vi "RateScan_Javi.vi"(0 "ftHandle_in":u32, 5 "VISA resource name":refnum<visa-resource-name>="USB0::0x0957::0x4108::MY51400415::INSTR", 7 "Path":path, 9 "String":string, 11 "error in (no error)":errorcluster) -> (4 "ftHandle_out":u32, 6 "VISA resource name out":refnum<visa-resource-name>, 15 "error out":errorcluster)   [LabVIEW 2019]
uses:
  Global_STOP.vi
  Library VI/Global.Salir Ya.vi
panel:
  out "B 2":u8(slide)=9 scale=0.0..100.0
  out "% 2":u8=9 format="%02d%%"
  out "Indicador 2":string="VTheo 0,0500V (Vreal 0,0000V)\nChannel 7 Adder C\nTotal Errors: 0"
  out "HLTHx 3":dbl
  out "DAC TH0,TH1,TH2 3":u16
  out "LLTHx 3":dbl
  out "DAC TH3,TH4,TH5 3":u16
  out "Reference 2":T1={"Sumador"=2, "Canal"=6, "Tension"=0, "Tension Real"=0.0}
  out "Amplitude 2":dbl
  out "B":u8(slide)=9 scale=0.0..100.0
  out "%":u8=9 format="%02d%%"
  out "Indicador":string="VTheo 0,0500V (Vreal 0,0000V)\nChannel 7 Adder C\nTotal Errors: 0"
  out "HLTHx 2":dbl
  out "DAC TH0,TH1,TH2 2":u16
  out "LLTHx 2":dbl
  out "DAC TH3,TH4,TH5 2":u16
  out "Reference":T1={"Sumador"=2, "Canal"=6, "Tension"=0, "Tension Real"=0.0}
  out "Amplitude":dbl
  out "EJECUTANDO TEST SUMADORES":u8(slide) scale=0.0..10.0
  out "Flag_programoPulso":bool
  out "spreadsheet string":string
  out "TOTAL VALORES LLTHX":dbl[][](array[numeric])
  out "Array":u16[](array[numeric])
  out "x*y":u32
  out "TOTAL VALORES HLTHX":dbl[][](array[numeric])
  out "Valor Asic":u16 format="%x"
  out "TOTAL VALORES":u16[][](array[numeric]) format="%x"
  out "DAC TH3,TH4,TH5":u16
  out "LLTHx":dbl
  out "DAC TH0,TH1,TH2":u16
  out "HLTHx":dbl
  # "IN"
  # "1 + 2 + 3"
  # "ADC"
  # "ADC"
  # "Vin Asic"
  # "Vin Asic"
  # "ADD A/1"
  # "ADD B/1"
  # "ADD C/1"
  # "ADD A/0"
  # "ADD B/0"
  # "ADD C/0"
  # "50mV"
  # "50mV"
  # "90mV"
  # "90mV"
  # "130mV"
  # "130mV"
  # "170mV"
  # "170mV"
  # "210mV"
  # "210mV"
  # "250mV"
  # "250mV"
  # "290mV"
  # "290mV"
  # "330mV"
  # "330mV"
  # "370mV"
  # "370mV"
  # "410mV"
  # "410mV"
  # "TH0"
  # "TH1"
  # "TH2"
  # "DAC"
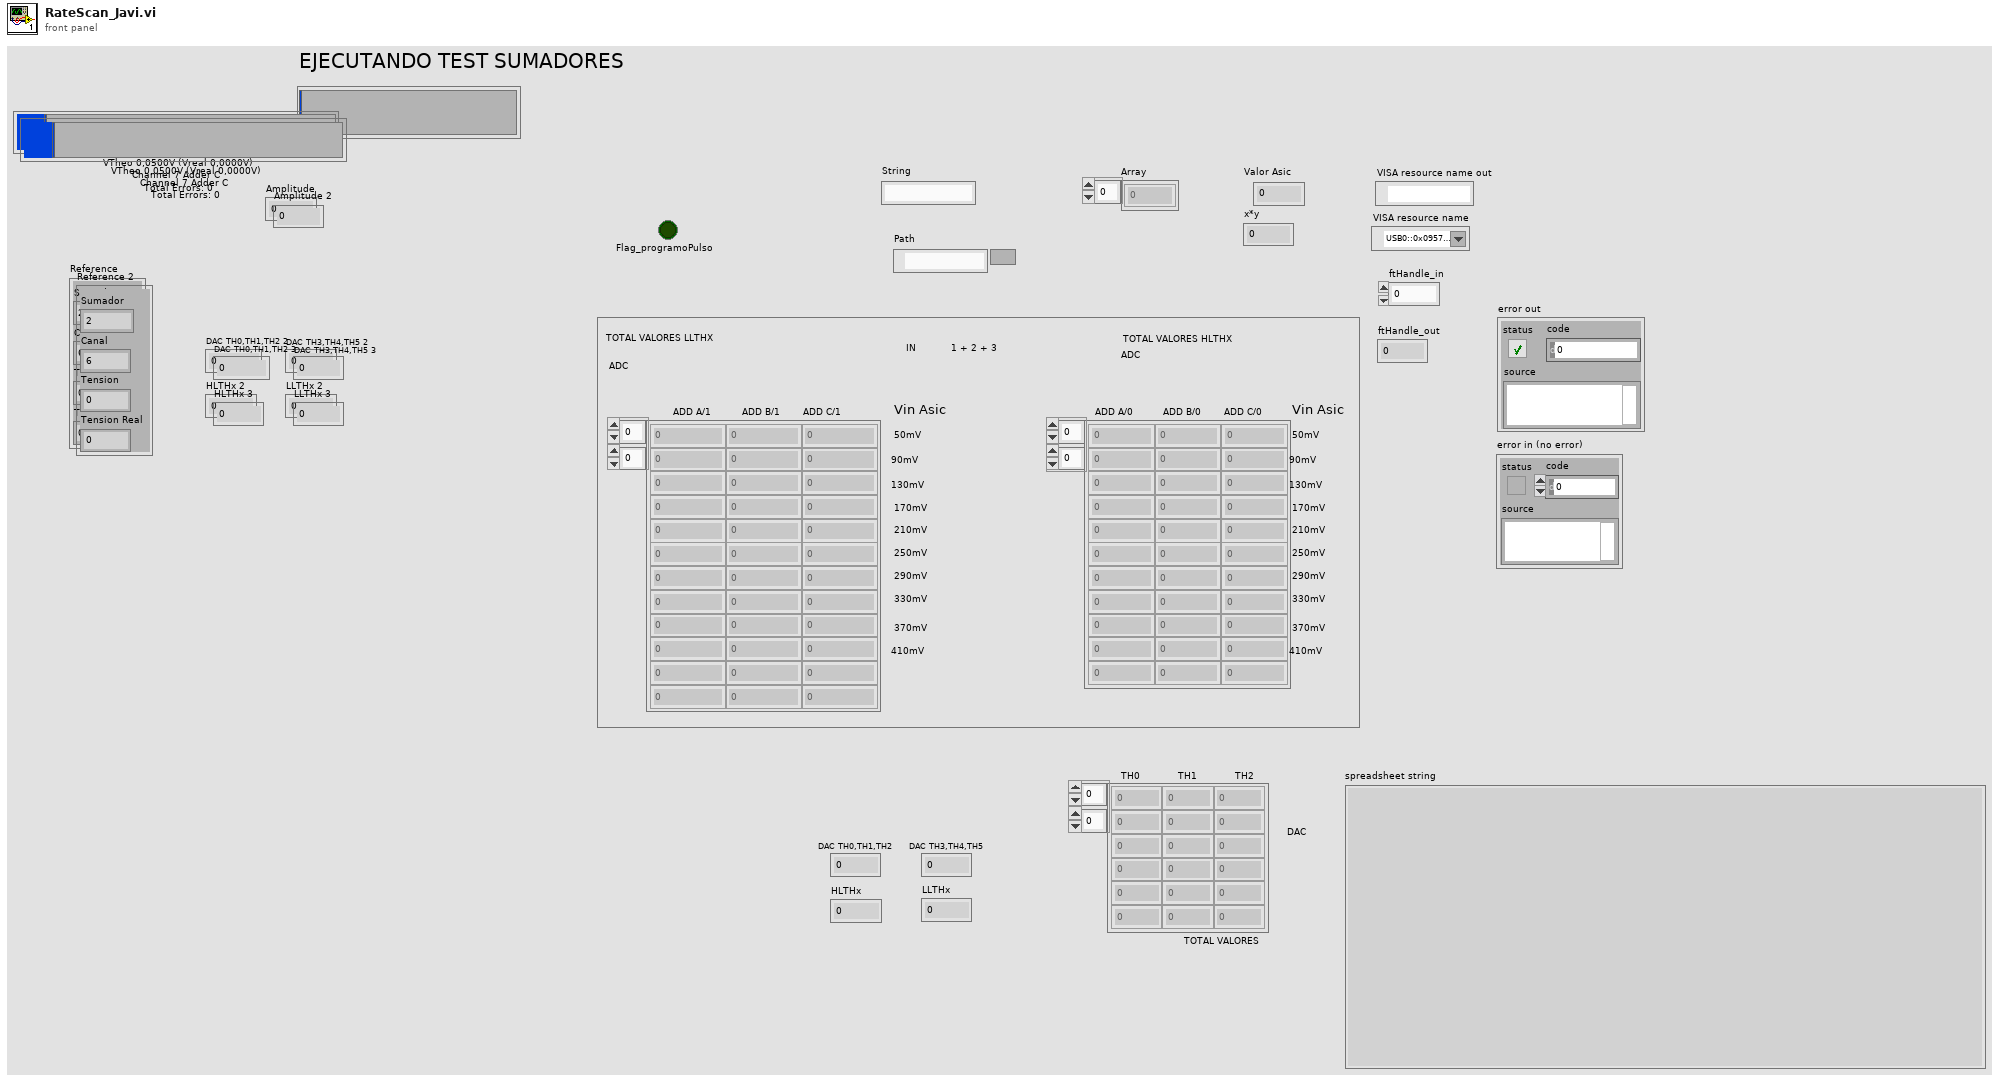
[diagram p1: front panel]
types:
  T1 = cluster{"Sumador":u8, "Canal":u8, "Tension":u8, "Tension Real":dbl}
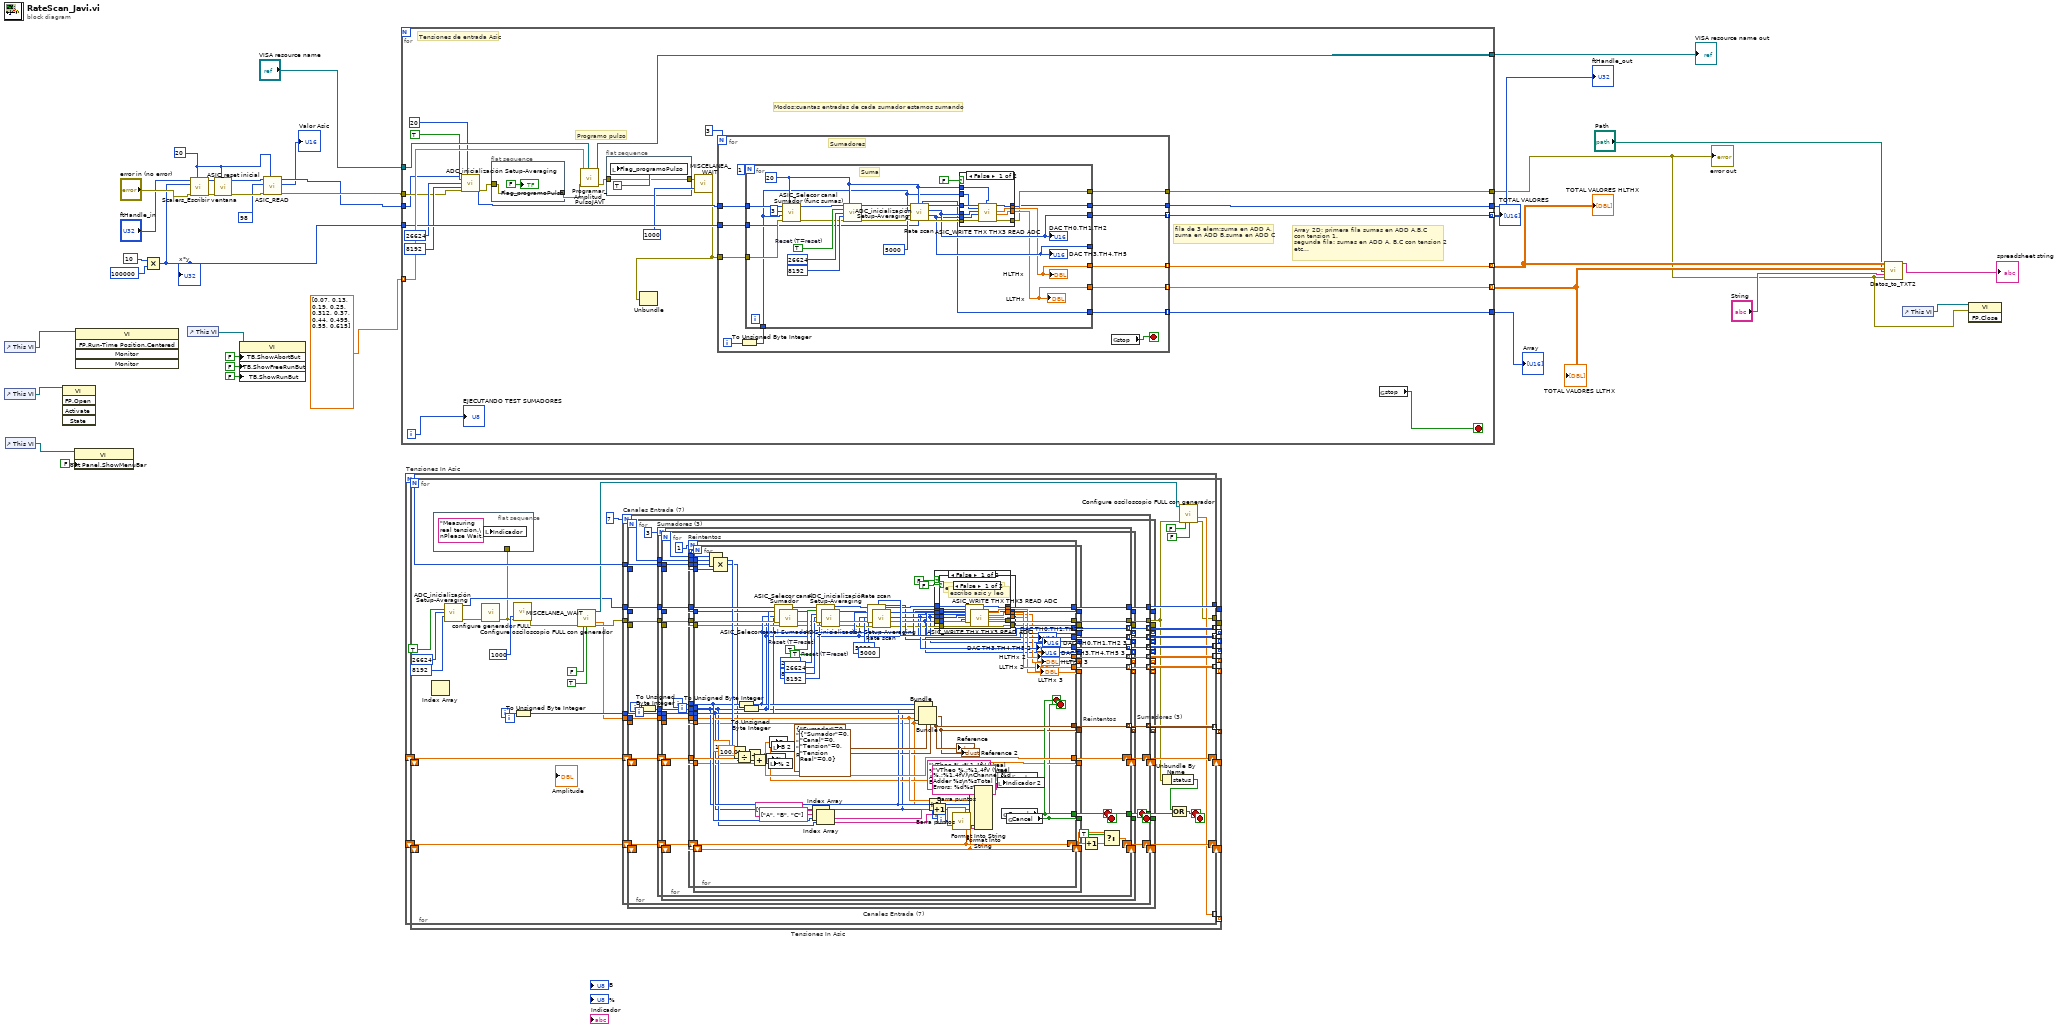
[diagram p0: block diagram]
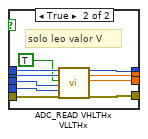
[diagram p2: hidden frame]
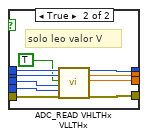
[diagram p3: hidden frame]
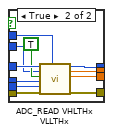
[diagram p4: hidden frame]
diagram:
  w18 = u32 20 ("Espera acceso USB")
  n1 = control-ref of="This VI"() -> (w10:refnum<vi>)
  n2 = control-ref of="This VI"() -> (w7:refnum<vi>)
  n3 = control-ref of="This VI"() -> (w6:refnum<vi>)
  n4 = invoke class="VI" method="FP.Open"(reference=w7) -> ()  [unwired: 4 in, 5 out]
  n5 = property class="VI"(reference=w6, "Front Panel.ShowMenuBar"=FALSE ("Front Panel Window:Show Menu Bar")) -> ()  [unwired: 1 in, 2 out]
  n6 = invoke class="VI" method="FP.Run-Time Position.Centered"(reference=w10) -> ()  [unwired: 4 in, 5 out]
  n7 = Multiply(x=u32 10 ("Ventana"), y=u32 100000 ("Ventana")) -> (x*y=w28:u32)
  "x*y" <- w28
  n8 = control-ref of="This VI"() -> (w4:refnum<vi>)
  n9 = call "Scalers_Escribir ventana.vi"("Espera acceso USB"=w18, "error in"="error in (no error)", "Ventana"=w28, "ftHandle_in"="ftHandle_in") -> ("error out"=w33:errorcluster, "ftHandle_out"=w32:u32)  [unwired: 6 in]
  n10 = call "ASIC_reset inicial.vi"("Espera acceso USB"=w18, "error in"=w33, "ftHandle_in"=w32) -> ("error out"=w23:errorcluster, "ftHandle_out"=w24:u32)  [unwired: 7 in]
  n11 = property class="VI"(reference=w4, "TB.ShowAbortBut"=FALSE ("Tool Bar:Show Abort Button"), "TB.ShowFreeRunBut"=FALSE ("Tool Bar:Show Free Run Button"), "TB.ShowRunBut"=FALSE ("Tool Bar:Show Run Button")) -> ()  [unwired: 1 in, 2 out]
  n12 = call "ASIC_READ.vi"("Espera acceso USB"=w18, "error in"=w23, "Direccion Registro Asic"=u8 98, "ftHandle_in"=w24) -> ("error out"=w22:errorcluster, "Valor Asic"=→"Valor Asic":u16, "ftHandle_out"=w21:u32)  [unwired: 5 in]
  n13 = for {
    tunnel: dbl[] [0.07, 0.13, 0.19, 0.25, 0.312, 0.37, 0.44, 0.495, 0.55, 0.615] -> [w61] mode=indexing
    tunnel: "VISA resource name" -> [w60]
    tunnel: w21 -> [w47]
    tunnel: w22 -> [w49]
    tunnel: w28 -> [w59]
    tunnel: [w58] -> w8
    tunnel: [w57] -> w27
    tunnel: [w56] -> w26
    tunnel: [w55] -> w25 mode=indexing
    tunnel: [w54] -> w17
    tunnel: [w44] -> w15 mode=indexing
    tunnel: [w43] -> w14 mode=indexing
    i -> [w36]
    stop <- w37 stop-if-true
    # "fila de 3 elem:suma en ADD A,\nsuma en ADD B,suma en ADD C"
    # "Modos:cuantas entradas de cada sumador estamos sumando"
    # "Array 2D: primera fila sumas en ADD A,B,C\ncon tension 1.\nsegunda fila: sumas en ADD A, B,C con tension 2\netc..."
    # "Programo pulso"
    # "Tensiones de entrada Asic"
    n14 = call "ADC_inicialización Setup-Averaging.vi"("ftHandle_in 2"=w47, "Espera acceso USB"=u32 20, "Reset (T=reset)"=TRUE, "Registro Setup (0x6800)"=u16 26624, "Registro Averaging (0x3200)"=u16 8192 ("Registro Setup (0x6800)"), "error in 2"=w49) -> ("ftHandle_out"=w46:u32, "error out"=w41:errorcluster)  [unwired: 8 in]
    n15 = flat-sequence {
      tunnel: [w65] -> w40
      tunnel: w41 -> [w65]
      frame #0 {
        "Flag_programoPulso" <- FALSE ("Flag_programoPulso")
      }
    }
    n16 = call "Programar_Amplitud_PulsoJAVI.vi"("error in (no error)"=w40, "Numeric"=w61, "VISA Refnum in"=w60) -> ("Error OUT"=w39:errorcluster, "VISA resource name out"=w57:refnum<visa-resource-name>)  [unwired: 7 in]
    n17 = flat-sequence {
      tunnel: w39 -> [w62]
      tunnel: [w62] -> w38
      frame #0 {
        n18 = local write "Flag_programoPulso"(TRUE ("Flag_programoPulso")) -> ()
      }
    }
    n19 = call "MISCELANEA_WAIT.vi"("ms wait IN"=u32 1000, "Error IN"=w38) -> ("Error OUT"=w42:errorcluster)  [unwired: 16 in, 1 out]
    n20 = Unbundle(w42) -> ()  [unwired: 3 out]
    n21 = for {
      N: 3 -> [_]
      tunnel: w46 -> [w77]
      tunnel: w42 -> [w74]
      tunnel: w59 -> [w73]
      tunnel: [w72] -> w55 mode=indexing
      tunnel: [w71] -> w58
      tunnel: [w70] -> w56
      tunnel: [w69] -> w54 mode=indexing
      tunnel: [w68] -> w44 mode=indexing
      tunnel: [w67] -> w43 mode=indexing
      i -> [w76]
      stop <- w66 stop-if-true
      # "Sumadores"
      n22 = To Unsigned Byte Integer(number=w76) -> (unsigned 8bit integer=w75:u8)
      n23 = for {
        N: 1 -> [_]
        tunnel: w77 -> [w91]
        tunnel: w75 -> [w80]
        tunnel: w74 -> [w90]
        tunnel: w73 -> [w88]
        tunnel: [w87] -> w72
        tunnel: [w86] -> _
        tunnel: [w85] -> w68
        tunnel: [w84] -> w67
        tunnel: [w83] -> w71
        tunnel: [w82] -> w69
        tunnel: [w81] -> w70
        w89 = u32 20 ("Espera acceso USB")
        w102 = TRUE  # Reset (T=reset)
        # "Suma"
        n24 = call "ASIC_Selecor canal Sumador (func sumas).vi"("Espera acceso USB"=w89, "error in"=w90, "Sumador"=w80, "Modo"=u8 3, "ftHandle_in"=w91) -> ("error out"=w97:errorcluster, "ftHandle_out"=w94:u32)  [unwired: 3 in, 2 out]
        n25 = call "ADC_inicialización Setup-Averaging.vi"("ftHandle_in 2"=w94, "Espera acceso USB"=w89, "Reset (T=reset)"=w102, "Registro Setup (0x6800)"=u16 26624, "Registro Averaging (0x3200)"=u16 8192 ("Registro Setup (0x6800)"), "error in 2"=w97) -> ("ftHandle_out"=w99:u32, "error out"=w98:errorcluster)  [unwired: 8 in]
        n26 = call "Rate scan.vi"("T Ventana"=w88, "Espera acceso USB"=w89, "error in 2"=w98, "Valor buscado scalers (5000)"=u16 5000 ("Valor buscado scalers"), "Sumador"=w80, "ftHandle_in 2"=w99) -> ("error out 2"=w95:errorcluster, "DAC\nTH3,TH4,TH5"=w86:u16, "DAC\nTH0,TH1,TH2"=w87:u16, "ftHandle_out 2"=w96:u32, "Scaler 1"=w82:u16)  [unwired: 1 in]
        "DAC TH0,TH1,TH2" <- w87
        "DAC TH3,TH4,TH5" <- w86
        n27 = case shown="False" FALSE {
          tunnel: w96 -> [w112 w123]
          tunnel: w95 -> [w109 w122]
          tunnel: [w107 w121] -> w81
          tunnel: [w108 w120] -> w83
          tunnel: [w106 w119] -> w85
          tunnel: [w105 w118] -> w84
          tunnel: w87 -> [w111 w117]
          tunnel: w86 -> [w110 w116]
          tunnel: w89 -> [w104 w114]
          tunnel: w80 -> [w103 w113]
          frame False {
            n28 = call "ASIC_WRITE THX THX3 READ ADC.vi"("ftHandle_in"=w112, "Sumador"=w103, "THX"=w111, "THX+3"=w110, "error in"=w109, "Espera acceso USB 2"=w104) -> ("ftHandle_out"=w107:u32, "HLTHx"=w106:dbl, "LLTHx"=w105:dbl, "error out"=w108:errorcluster)  [unwired: 10 in]
          }
          frame True {
            n29 = call "ADC_READ VHLTHx VLLTHx.vi"("ftHandle_out 2"=w123, "Sumador"=w113, "referenciar"=TRUE, "ref DAC\nTH0,TH1,TH2"=w117, "ref DAC\nTH3,TH4,TH5"=w116, "error out 2"=w122, "Espera acceso FT"=w114) -> ("ftHandle_out"=w121:u32, "HLTHx"=w119:dbl, "LLTHx"=w118:dbl, "error out"=w120:errorcluster)  [unwired: 9 in]
          }
        }
        "HLTHx" <- w85
        "LLTHx" <- w84
      }
      n30 = global read "Global_STOP.vi" "stop"() -> (w66:bool)
    }
    n31 = global read "Global_STOP.vi" "stop"() -> (w37:bool)
    "EJECUTANDO TEST SUMADORES" <- w36
  }
  "error out" <- w8
  "VISA resource name out" <- w27
  "ftHandle_out" <- w26
  "TOTAL VALORES" <- w25
  "TOTAL VALORES HLTHX" <- w15
  "Array" <- w17
  "TOTAL VALORES LLTHX" <- w14
  n32 = for "Tensiones In Asic" {
    N -> [w146]
    tunnel: [w157] -> _ mode=indexing
    tunnel: [w156] -> _ mode=indexing
    tunnel: [w152] -> _ mode=indexing
    tunnel: [w151] -> _ mode=indexing
    tunnel: [w149] -> _ mode=indexing
    tunnel: [w147] -> _ mode=indexing
    shift-right: [w144] -> _
    shift-left: _ -> [w145]
    shift-right: [w142] -> _
    shift-left: _ -> [w143]
    tunnel: [w158] -> _
    tunnel: [w135] -> _
    tunnel: [w136] -> _ mode=indexing
    i -> [w150]
    stop <- w127 stop-if-true
    n33 = Index Array() -> ()  [unwired: 2 in, 1 out]
    n34 = flat-sequence {
      tunnel: w124 -> [_]
      frame #0 {
        n35 = local write "Indicador"("Measuring real tension.\nPlease Wait." ("Indicador")) -> ()
      }
    }
    n36 = call "ADC_inicialización Setup-Averaging.vi"("Reset (T=reset)"=TRUE, "Registro Setup (0x6800)"=u16 26624, "Registro Averaging (0x3200)"=u16 8192 ("Registro Setup (0x6800)")) -> ("ftHandle_out"=w126:u32, "error out"=w125:errorcluster)  [unwired: 11 in]
    n37 = call "configure generador FULL.vi"("error in"=w125) -> ("error out"=w124:errorcluster)  [unwired: 8 in, 2 out]
    n38 = call "MISCELANEA_WAIT.vi"("ms wait IN"=u32 1000, "Error IN"=w124) -> ("Error OUT"=w140:errorcluster)  [unwired: 16 in, 1 out]
    n39 = To Unsigned Byte Integer(number=w150) -> (unsigned 8bit integer=w148:u8)
    n40 = call "Configure osciloscopio FULL con generador.vi"("error out"=w140, "Esperar a completar estadisticas"=FALSE ("Wait medida"), "Configurar Osciloscopio"=TRUE ("Solo Medida")) -> ("VISA resource name out 2"=w131:refnum<visa-resource-name>, "Math (CH1-CH2)"=w137:dbl, "error out 2"=w139:errorcluster)  [unwired: 8 in, 2 out]
    n41 = for "Canales Entrada (7)" {
      N: 7 -> [w167]
      tunnel: [w175] -> w157 mode=indexing
      tunnel: [w174] -> w156 mode=indexing
      tunnel: [w173] -> w152 mode=indexing
      tunnel: [w172] -> w151 mode=indexing
      tunnel: w148 -> [w171]
      tunnel: w137 -> [w170]
      tunnel: [w169] -> w149 mode=indexing
      tunnel: [w168] -> w147 mode=indexing
      tunnel: w146 -> [w166]
      shift-right: [w164] -> w144
      shift-left: w145 -> [w165]
      tunnel: [w163] -> w128
      shift-right: [w161] -> w142
      shift-left: w143 -> [w162]
      tunnel: w126 -> [w182]
      tunnel: [w177] -> w158
      tunnel: w139 -> [w181]
      tunnel: [w176] -> w130
      i -> [w180]
      stop <- w163 stop-if-true
      n42 = To Unsigned Byte Integer(number=w180) -> (unsigned 8bit integer=w178:u8)
      n43 = for "Sumadores (3)" {
        N: 3 -> [w200]
        tunnel: w178 -> [w196]
        tunnel: [w208] -> w175 mode=indexing
        tunnel: [w207] -> w174 mode=indexing
        tunnel: [w192] -> w173 mode=indexing
        tunnel: [w191] -> w172 mode=indexing
        tunnel: w171 -> [w201]
        tunnel: w170 -> [w197]
        tunnel: [w203] -> w169 mode=indexing
        tunnel: [w202] -> w168 mode=indexing
        tunnel: w167 -> [w199]
        tunnel: w166 -> [w198]
        shift-right: [w193] -> w164
        shift-left: w165 -> [w194]
        tunnel: [w188] -> w163
        shift-right: [w187] -> w161
        shift-left: w162 -> [w189]
        tunnel: w182 -> [w205]
        tunnel: [w204] -> w177
        tunnel: w181 -> [w206]
        tunnel: [w183] -> w176
        i -> [w195]
        stop <- w188 stop-if-true
        n44 = for "Reintentos" {
          N: 1 -> [_]
          tunnel: [w215] -> w208
          tunnel: [w214] -> w207
          tunnel: w205 -> [w249]
          tunnel: [w246] -> w204
          tunnel: [w243] -> w203
          tunnel: [w242] -> w202
          tunnel: w201 -> [w221]
          tunnel: w200 -> [w240]
          tunnel: w199 -> [w239]
          tunnel: w198 -> [w238]
          tunnel: w197 -> [w209]
          tunnel: w196 -> [w212]
          tunnel: w195 -> [w234]
          tunnel: [w210] -> w188
          tunnel: [w226] -> w192
          tunnel: [w225] -> w191
          tunnel: w194 -> [w229]
          tunnel: [w227] -> w193
          shift-right: [w222] -> w186
          shift-left: w189 -> [w222]
          tunnel: w206 -> [w250]
          tunnel: [w245] -> w183
          i -> [w224]
          stop <- w210 stop-if-true
          w252 = TRUE  # Reset (T=reset)
          n45 = for "Tensiones In Asic" {
            N -> [w275]
            tunnel: [w286] -> _ mode=indexing
            tunnel: [w285] -> _ mode=indexing
            tunnel: [w281] -> _ mode=indexing
            tunnel: [w280] -> _ mode=indexing
            tunnel: [w278] -> _ mode=indexing
            tunnel: [w276] -> _ mode=indexing
            shift-right: [w273] -> _
            shift-left: _ -> [w274]
            shift-right: [w271] -> _
            shift-left: _ -> [w272]
            tunnel: [w287] -> _
            tunnel: [w264] -> _
            tunnel: [w265] -> _ mode=indexing
            i -> [w279]
            stop <- w256 stop-if-true
            n46 = Index Array() -> ()  [unwired: 2 in, 1 out]
            n47 = flat-sequence {
              tunnel: w253 -> [_]
              frame #0 {
                n48 = local write "Indicador 2"("Measuring real tension.\nPlease Wait." ("Indicador")) -> ()
              }
            }
            n49 = call "ADC_inicialización Setup-Averaging.vi"("Reset (T=reset)"=TRUE, "Registro Setup (0x6800)"=u16 26624, "Registro Averaging (0x3200)"=u16 8192 ("Registro Setup (0x6800)")) -> ("ftHandle_out"=w255:u32, "error out"=w254:errorcluster)  [unwired: 11 in]
            n50 = call "configure generador FULL.vi"("error in"=w254) -> ("error out"=w253:errorcluster)  [unwired: 8 in, 2 out]
            n51 = call "MISCELANEA_WAIT.vi"("ms wait IN"=u32 1000, "Error IN"=w253) -> ("Error OUT"=w269:errorcluster)  [unwired: 16 in, 1 out]
            n52 = To Unsigned Byte Integer(number=w279) -> (unsigned 8bit integer=w277:u8)
            n53 = call "Configure osciloscopio FULL con generador.vi"("error out"=w269, "Esperar a completar estadisticas"=FALSE ("Wait medida"), "Configurar Osciloscopio"=TRUE ("Solo Medida")) -> ("VISA resource name out 2"=w260:refnum<visa-resource-name>, "Math (CH1-CH2)"=w266:dbl, "error out 2"=w268:errorcluster)  [unwired: 8 in, 2 out]
            n54 = for "Canales Entrada (7)" {
              N: 7 -> [w296]
              tunnel: [w304] -> w286 mode=indexing
              tunnel: [w303] -> w285 mode=indexing
              tunnel: [w302] -> w281 mode=indexing
              tunnel: [w301] -> w280 mode=indexing
              tunnel: w277 -> [w300]
              tunnel: w266 -> [w299]
              tunnel: [w298] -> w278 mode=indexing
              tunnel: [w297] -> w276 mode=indexing
              tunnel: w275 -> [w295]
              shift-right: [w293] -> w273
              shift-left: w274 -> [w294]
              tunnel: [w292] -> w257
              shift-right: [w290] -> w271
              shift-left: w272 -> [w291]
              tunnel: w255 -> [w311]
              tunnel: [w306] -> w287
              tunnel: w268 -> [w310]
              tunnel: [w305] -> w259
              i -> [w309]
              stop <- w292 stop-if-true
              n55 = To Unsigned Byte Integer(number=w309) -> (unsigned 8bit integer=w307:u8)
              n56 = for "Sumadores (3)" {
                N: 3 -> [w329]
                tunnel: w307 -> [w325]
                tunnel: [w337] -> w304 mode=indexing
                tunnel: [w336] -> w303 mode=indexing
                tunnel: [w321] -> w302 mode=indexing
                tunnel: [w320] -> w301 mode=indexing
                tunnel: w300 -> [w330]
                tunnel: w299 -> [w326]
                tunnel: [w332] -> w298 mode=indexing
                tunnel: [w331] -> w297 mode=indexing
                tunnel: w296 -> [w328]
                tunnel: w295 -> [w327]
                shift-right: [w322] -> w293
                shift-left: w294 -> [w323]
                tunnel: [w317] -> w292
                shift-right: [w316] -> w290
                shift-left: w291 -> [w318]
                tunnel: w311 -> [w334]
                tunnel: [w333] -> w306
                tunnel: w310 -> [w335]
                tunnel: [w312] -> w305
                i -> [w324]
                stop <- w317 stop-if-true
                n57 = for "Reintentos" {
                  N: 1 -> [_]
                  tunnel: [w344] -> w337
                  tunnel: [w343] -> w336
                  tunnel: w334 -> [w378]
                  tunnel: [w375] -> w333
                  tunnel: [w372] -> w332
                  tunnel: [w371] -> w331
                  tunnel: w330 -> [w350]
                  tunnel: w329 -> [w369]
                  tunnel: w328 -> [w368]
                  tunnel: w327 -> [w367]
                  tunnel: w326 -> [w338]
                  tunnel: w325 -> [w341]
                  tunnel: w324 -> [w363]
                  tunnel: [w339] -> w317
                  tunnel: [w355] -> w321
                  tunnel: [w354] -> w320
                  tunnel: w323 -> [w358]
                  tunnel: [w356] -> w322
                  shift-right: [w351] -> w315
                  shift-left: w318 -> [w351]
                  tunnel: w335 -> [w379]
                  tunnel: [w374] -> w312
                  i -> [w353]
                  stop <- w339 stop-if-true
                  w381 = TRUE  # Reset (T=reset)
                  n58 = Compound Arithmetic op=MULTIPLY(w369, w368, w367) -> (w366:i32)
                  n59 = Divide(x=100.0, y=w366) -> (x/y=w357:dbl)
                  n60 = To Unsigned Byte Integer(number=w363) -> (unsigned 8bit integer=w340:u8)
                  n61 = Add(x=w357, y=w358) -> (x+y=w356:dbl)
                  n62 = local write "% 2"(w356) -> ()
                  n63 = local write "B 2"(w356) -> ()
                  n64 = call "ASIC_Selecor canal Sumador.vi"("error in"=w379, "Sumador"=w340, "Canal"=w341, "ftHandle_in"=w378) -> ("error out"=w377:errorcluster, "ftHandle_out"=w376:u32)  [unwired: 5 in, 1 out]
                  n65 = Index Array(array=string[] ["A", "B", "C"], index=w363) -> (element=w362:string)
                  n66 = call "ADC_inicialización Setup-Averaging.vi"("ftHandle_in 2"=w376, "Reset (T=reset)"=w381, "Registro Setup (0x6800)"=u16 26624, "Registro Averaging (0x3200)"=u16 8192 ("Registro Setup (0x6800)"), "error in 2"=w377) -> ("ftHandle_out"=w349:u32, "error out"=w348:errorcluster)  [unwired: 9 in]
                  n67 = call "Rate scan.vi"("error in 2"=w348, "Valor buscado scalers (5000)"=u16 5000 ("Valor buscado scalers"), "Sumador"=w340, "ftHandle_in 2"=w349) -> ("error out 2"=w346:errorcluster, "DAC\nTH3,TH4,TH5"=w343:u16, "DAC\nTH0,TH1,TH2"=w344:u16, "ftHandle_out 2"=w347:u32, "Scaler 1"=w372:u16)  [unwired: 3 in]
                  "DAC TH0,TH1,TH2 3" <- w344
                  "DAC TH3,TH4,TH5 3" <- w343
                  n68 = Bundle(cluster=T1 {"Sumador"=0, "Canal"=0, "Tension"=0, "Tension Real"=0.0}, "Sumador"=w340, "Canal"=w341, "Tension"=w350, "Tension Real"=w338) -> (w371:T1)
                  "Reference 2" <- w371
                  n69 = Increment(x=w341) -> (x+1=w360:u8)
                  n70 = case shown="False" FALSE {
                    tunnel: [w390 w400] -> w375
                    tunnel: [w384 w399] -> w374
                    tunnel: [w382 w398] -> w355
                    tunnel: [w383 w397] -> w354
                    tunnel: w340 -> [w388 w396]
                    tunnel: w347 -> [w389 w395]
                    tunnel: w346 -> [w385 w394]
                    tunnel: w344 -> [w387 w393]
                    tunnel: w343 -> [w386 w392]
                    frame False {
                      # "escribo asic y leo"
                      n71 = call "ASIC_WRITE THX THX3 READ ADC.vi"("ftHandle_in"=w389, "Sumador"=w388, "THX"=w387, "THX+3"=w386, "error in"=w385) -> ("ftHandle_out"=w390:u32, "HLTHx"=w382:dbl, "LLTHx"=w383:dbl, "error out"=w384:errorcluster)  [unwired: 11 in]
                    }
                    frame True {
                      # "solo leo valor V"
                      n72 = call "ADC_READ VHLTHx VLLTHx.vi"("ftHandle_out 2"=w395, "Sumador"=w396, "referenciar"=TRUE, "ref DAC\nTH0,TH1,TH2"=w393, "ref DAC\nTH3,TH4,TH5"=w392, "error out 2"=w394) -> ("ftHandle_out"=w400:u32, "HLTHx"=w398:dbl, "LLTHx"=w397:dbl, "error out"=w399:errorcluster)  [unwired: 10 in]
                    }
                  }
                  "HLTHx 3" <- w355
                  "LLTHx 3" <- w354
                  n73 = call "Barra puntos.vi"("#N"=w353) -> ("String"=w352:string)  [unwired: 8 in]
                  n74 = Format Into String(format string="VTheo %,;%1.4fV (Vreal %,;%1.4fV)\nChannel %d Adder %s\n%sTotal Errors: %d%s", w338, w360, w362, w352, w351, w352) -> (resulting string=w361:string)  [unwired: 3 in, 1 out]
                  n75 = local write "Indicador 2"(w361) -> ()
                  n76 = global read "Global.Salir Ya.vi" "Cancel"() -> (w339:bool)
                }
                n77 = Increment(x=w315) -> (x+1=w314:dbl)
                n78 = Select(t=w315, s=TRUE, f=w314) -> (s? t:f=w316:dbl)
              }
            }
            n79 = Unbundle By Name(w259) -> ("status"=w258:bool)
            n80 = Compound Arithmetic op=OR(w258, w257) -> (w256:bool)
            n81 = call "Configure osciloscopio FULL con generador.vi"("Visa MDO3104"=w260, "error out"=w259, "Esperar a completar estadisticas"=FALSE, "Configurar Osciloscopio"=FALSE ("Solo Medida")) -> ("Math (CH1-CH2)"=w265:dbl, "error out 2"=w264:errorcluster)  [unwired: 7 in, 3 out]
          }
          n82 = Compound Arithmetic op=MULTIPLY(w240, w239, w238) -> (w237:i32)
          n83 = Divide(x=100.0, y=w237) -> (x/y=w228:dbl)
          n84 = To Unsigned Byte Integer(number=w234) -> (unsigned 8bit integer=w211:u8)
          n85 = Add(x=w228, y=w229) -> (x+y=w227:dbl)
          n86 = local write "%"(w227) -> ()
          n87 = local write "B"(w227) -> ()
          n88 = call "ASIC_Selecor canal Sumador.vi"("error in"=w250, "Sumador"=w211, "Canal"=w212, "ftHandle_in"=w249) -> ("error out"=w248:errorcluster, "ftHandle_out"=w247:u32)  [unwired: 5 in, 1 out]
          n89 = Index Array(array=string[] ["A", "B", "C"], index=w234) -> (element=w233:string)
          n90 = call "ADC_inicialización Setup-Averaging.vi"("ftHandle_in 2"=w247, "Reset (T=reset)"=w252, "Registro Setup (0x6800)"=u16 26624, "Registro Averaging (0x3200)"=u16 8192 ("Registro Setup (0x6800)"), "error in 2"=w248) -> ("ftHandle_out"=w220:u32, "error out"=w219:errorcluster)  [unwired: 9 in]
          n91 = call "Rate scan.vi"("error in 2"=w219, "Valor buscado scalers (5000)"=u16 5000 ("Valor buscado scalers"), "Sumador"=w211, "ftHandle_in 2"=w220) -> ("error out 2"=w217:errorcluster, "DAC\nTH3,TH4,TH5"=w214:u16, "DAC\nTH0,TH1,TH2"=w215:u16, "ftHandle_out 2"=w218:u32, "Scaler 1"=w243:u16)  [unwired: 3 in]
          "DAC TH0,TH1,TH2 2" <- w215
          "DAC TH3,TH4,TH5 2" <- w214
          n92 = Bundle(cluster=T1 {"Sumador"=0, "Canal"=0, "Tension"=0, "Tension Real"=0.0}, "Sumador"=w211, "Canal"=w212, "Tension"=w221, "Tension Real"=w209) -> (w242:T1)
          "Reference" <- w242
          n93 = Increment(x=w212) -> (x+1=w231:u8)
          n94 = case shown="False" FALSE {
            tunnel: [w409 w419] -> w246
            tunnel: [w403 w418] -> w245
            tunnel: [w401 w417] -> w226
            tunnel: [w402 w416] -> w225
            tunnel: w211 -> [w407 w415]
            tunnel: w218 -> [w408 w414]
            tunnel: w217 -> [w404 w413]
            tunnel: w215 -> [w406 w412]
            tunnel: w214 -> [w405 w411]
            frame False {
              # "escribo asic y leo"
              n95 = call "ASIC_WRITE THX THX3 READ ADC.vi"("ftHandle_in"=w408, "Sumador"=w407, "THX"=w406, "THX+3"=w405, "error in"=w404) -> ("ftHandle_out"=w409:u32, "HLTHx"=w401:dbl, "LLTHx"=w402:dbl, "error out"=w403:errorcluster)  [unwired: 11 in]
            }
            frame True {
              # "solo leo valor V"
              n96 = call "ADC_READ VHLTHx VLLTHx.vi"("ftHandle_out 2"=w414, "Sumador"=w415, "referenciar"=TRUE, "ref DAC\nTH0,TH1,TH2"=w412, "ref DAC\nTH3,TH4,TH5"=w411, "error out 2"=w413) -> ("ftHandle_out"=w419:u32, "HLTHx"=w417:dbl, "LLTHx"=w416:dbl, "error out"=w418:errorcluster)  [unwired: 10 in]
            }
          }
          "HLTHx 2" <- w226
          "LLTHx 2" <- w225
          n97 = call "Barra puntos.vi"("#N"=w224) -> ("String"=w223:string)  [unwired: 8 in]
          n98 = Format Into String(format string="VTheo %,;%1.4fV (Vreal %,;%1.4fV)\nChannel %d Adder %s\n%sTotal Errors: %d%s", w209, w231, w233, w223, w222, w223) -> (resulting string=w232:string)  [unwired: 3 in, 1 out]
          n99 = local write "Indicador"(w232) -> ()
          n100 = global read "Global.Salir Ya.vi" "Cancel"() -> (w210:bool)
        }
        n101 = Increment(x=w186) -> (x+1=w185:dbl)
        n102 = Select(t=w186, s=TRUE, f=w185) -> (s? t:f=w187:dbl)
      }
    }
    n103 = Unbundle By Name(w130) -> ("status"=w129:bool)
    n104 = Compound Arithmetic op=OR(w129, w128) -> (w127:bool)
    n105 = call "Configure osciloscopio FULL con generador.vi"("Visa MDO3104"=w131, "error out"=w130, "Esperar a completar estadisticas"=FALSE, "Configurar Osciloscopio"=FALSE ("Solo Medida")) -> ("Math (CH1-CH2)"=w136:dbl, "error out 2"=w135:errorcluster)  [unwired: 7 in, 3 out]
  }
  n106 = call "Datos_to_TXT2.vi"("Array"=w15, "Array 2"=w14, "Path"="Path", "String"="String", "error in (no error)"=w8) -> ("spreadsheet string"=→"spreadsheet string":string)  [unwired: 10 in]
  n107 = control-ref of="This VI"() -> (w9:refnum<vi>)
  n108 = invoke class="VI" method="FP.Close"(reference=w9, error in=w8) -> ()  [unwired: 1 in, 3 out]
